vi "Exit.vi"(8 "error in (no error)":errorcluster, 11 "Old State":refnum<class "Command.lvclass">) -> (0 "error out":errorcluster, 3 "New State":refnum<class "Command.lvclass">)   [LabVIEW 2013, in "Command Processor.lvlib" / "Command.lvlib" / "Command.lvclass"]
doc: "This is an abstract method. Override this method to define the behavior when you leave the state."
uses:
  Command.lvclass
  <vilib>/ni/Actors/State Actor/State Actor/State Actor.lvclass
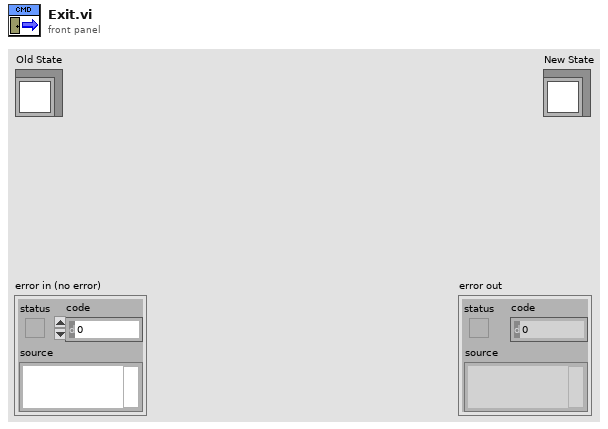
[diagram p1: front panel]
types:
  T1 = typedef "Command Processor.lvlib/Command.lvlib/Command.lvclass/Command Status.ctl" = cluster{"Command Name":string, "Current State Status":T2, "Command Start Time":timestamp, "Command End Time":timestamp, "Previous State Status":T2}
  T2 = typedef "Command Processor.lvlib/Command.lvlib/Command.lvclass/State Status.ctl" = cluster{"State Name":string, "State Entry Time":timestamp, "State Exit Time":timestamp}
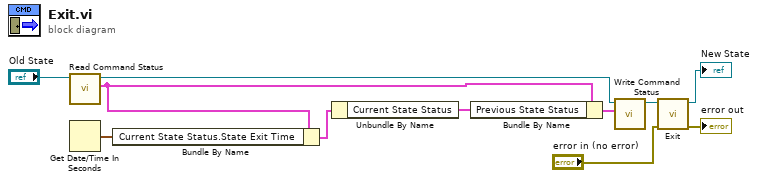
[diagram p0: block diagram]
diagram:
  n1 = call-dynamic "Read Command Status.vi"("Command in"="Old State") -> ("Command Status"=w5:T1, "Command out"=w8:refnum<class "Command.lvclass">)  [unwired: 8 in, 1 out]
  n2 = Get Date/Time In Seconds() -> (seconds since 1Jan1904=w1:timestamp)
  n3 = Bundle By Name(cluster=w5, "Current State Status.State Exit Time"=w1) -> (w2:T1)
  n4 = Unbundle By Name(w2) -> ("Current State Status"=w3:T2)
  n5 = Bundle By Name(cluster=w5, "Previous State Status"=w3) -> (w4:T1)
  n6 = call-dynamic "Write Command Status.vi"("Command Status"=w4, "Command in"=w8) -> ("Command out"=w6:refnum<class "Command.lvclass">)  [unwired: 8 in, 1 out]
  n7 = call-parent "Exit.vi"("error in (no error)"="error in (no error)", "Old State"=w6) -> ("error out"=→"error out":errorcluster, "New State"=→"New State":refnum<class "Command.lvclass">)  [unwired: 8 in]
